vi "CT_DischargeEntryCleanup.vi"(2 "Load Number":i32, 3 "Cap Discharge Array In":T1=[{"cap number and switch SN array"=[{"Switch SN"="SN_U", "Cap Number"=109.0}], "Rog"=enum."F240", "Delay"=enum."PreForm", "Power Supply"=enum."PS1"}, {"cap number and switch SN array"=[{"Switch SN"="SN_U", "Cap Number"=110.0}], "Rog"=enum."F180", "Delay"=enum."DB16", "Power Supply"=enum."PS2"}, {"cap number and switch SN array"=[{"Switch SN"="SN_U", "Cap Number"=111.0}], "Rog"=enum."F300", "Delay"=enum."DB16", "Power Supply"=enum."PS2"}, {"cap number and switch SN array"=[{"Switch SN"="SN_U", "Cap Number"=112.0}], "Rog"=enum."F000", "Delay"=enum."DB16", "Power Supply"=enum."PS2"}, {"cap number and switch SN array"=[{"Switch SN"="SN_U", "Cap Number"=113.0}], "Rog"=enum."F060", "Delay"=enum."DB16", "Power Supply"=enum."PS2"}, {"cap number and switch SN array"=[{"Switch SN"="SN_U", "Cap Number"=114.0}], "Rog"=enum."F120", "Delay"=enum."DB16", "Power Supply"=enum."PS2"}, {"cap number and switch SN array"=[{"Switch SN"="SN_U", "Cap Number"=115.0}], "Rog"=enum."F120", "Delay"=enum."DB16", "Power Supply"=enum."PS2"}, {"cap number and switch SN array"=[{"Switch SN"="SN_U", "Cap Number"=116.0}], "Rog"=enum."F060", "Delay"=enum."DB16", "Power Supply"=enum."PS2"}, {"cap number and switch SN array"=[{"Switch SN"="SN_U", "Cap Number"=117.0}], "Rog"=enum."F000", "Delay"=enum."DB16", "Power Supply"=enum."PS2"}, {"cap number and switch SN array"=[{"Switch SN"="SN_U", "Cap Number"=118.0}], "Rog"=enum."F300", "Delay"=enum."DB16", "Power Supply"=enum."PS2"}, {"cap number and switch SN array"=[{"Switch SN"="SN_U", "Cap Number"=119.0}], "Rog"=enum."F180", "Delay"=enum."DB16", "Power Supply"=enum."PS2"}, {"cap number and switch SN array"=[{"Switch SN"="SN_U", "Cap Number"=120.0}], "Rog"=enum."F240", "Delay"=enum."DB16", "Power Supply"=enum."PS2"}, {"cap number and switch SN array"=[{"Switch SN"="SN_U", "Cap Number"=121.0}], "Rog"=enum."F240", "Delay"=enum."DB16", "Power Supply"=enum."PS3"}, {"cap number and switch SN array"=[{"Switch SN"="SN_U", "Cap Number"=122.0}], "Rog"=enum."F300", "Delay"=enum."DB16", "Power Supply"=enum."PS3"}, {"cap number and switch SN array"=[{"Switch SN"="SN_U", "Cap Number"=123.0}], "Rog"=enum."F180", "Delay"=enum."DB16", "Power Supply"=enum."PS3"}, {"cap number and switch SN array"=[{"Switch SN"="SN_U", "Cap Number"=124.0}], "Rog"=enum."F240", "Delay"=enum."DB16", "Power Supply"=enum."PS3"}, {"cap number and switch SN array"=[{"Switch SN"="SN_U", "Cap Number"=125.0}], "Rog"=enum."DISC", "Delay"=enum."DB16", "Power Supply"=enum."PS3"}, {"cap number and switch SN array"=[{"Switch SN"="SN_U", "Cap Number"=126.0}], "Rog"=enum."F000", "Delay"=enum."DB16", "Power Supply"=enum."PS3"}, {"cap number and switch SN array"=[{"Switch SN"="SN_U", "Cap Number"=127.0}], "Rog"=enum."F060", "Delay"=enum."DB16", "Power Supply"=enum."PS3"}, {"cap number and switch SN array"=[{"Switch SN"="SN_U", "Cap Number"=128.0}], "Rog"=enum."DISC", "Delay"=enum."DB16", "Power Supply"=enum."PS3"}]) -> (0 "Index of Module":u32, 1 "Cap Discharge Array Out":T1=[{"cap number and switch SN array"=[{"Switch SN"="SN_U", "Cap Number"=109.0}], "Rog"=enum."F240", "Delay"=enum."PreForm", "Power Supply"=enum."PS1"}, {"cap number and switch SN array"=[{"Switch SN"="SN_U", "Cap Number"=110.0}], "Rog"=enum."F180", "Delay"=enum."DB16", "Power Supply"=enum."PS2"}, {"cap number and switch SN array"=[{"Switch SN"="SN_U", "Cap Number"=111.0}], "Rog"=enum."F300", "Delay"=enum."DB16", "Power Supply"=enum."PS2"}, {"cap number and switch SN array"=[{"Switch SN"="SN_U", "Cap Number"=112.0}], "Rog"=enum."F000", "Delay"=enum."DB16", "Power Supply"=enum."PS2"}, {"cap number and switch SN array"=[{"Switch SN"="SN_U", "Cap Number"=113.0}], "Rog"=enum."F060", "Delay"=enum."DB16", "Power Supply"=enum."PS2"}, {"cap number and switch SN array"=[{"Switch SN"="SN_U", "Cap Number"=114.0}], "Rog"=enum."F120", "Delay"=enum."DB16", "Power Supply"=enum."PS2"}, {"cap number and switch SN array"=[{"Switch SN"="SN_U", "Cap Number"=115.0}], "Rog"=enum."F120", "Delay"=enum."DB16", "Power Supply"=enum."PS2"}, {"cap number and switch SN array"=[{"Switch SN"="SN_U", "Cap Number"=116.0}], "Rog"=enum."F060", "Delay"=enum."DB16", "Power Supply"=enum."PS2"}, {"cap number and switch SN array"=[{"Switch SN"="SN_U", "Cap Number"=117.0}], "Rog"=enum."F000", "Delay"=enum."DB16", "Power Supply"=enum."PS2"}, {"cap number and switch SN array"=[{"Switch SN"="SN_U", "Cap Number"=118.0}], "Rog"=enum."F300", "Delay"=enum."DB16", "Power Supply"=enum."PS2"}, {"cap number and switch SN array"=[{"Switch SN"="SN_U", "Cap Number"=119.0}], "Rog"=enum."F180", "Delay"=enum."DB16", "Power Supply"=enum."PS2"}, {"cap number and switch SN array"=[{"Switch SN"="SN_U", "Cap Number"=120.0}], "Rog"=enum."F240", "Delay"=enum."DB16", "Power Supply"=enum."PS2"}, {"cap number and switch SN array"=[{"Switch SN"="SN_U", "Cap Number"=121.0}], "Rog"=enum."F240", "Delay"=enum."DB16", "Power Supply"=enum."PS3"}, {"cap number and switch SN array"=[{"Switch SN"="SN_U", "Cap Number"=122.0}], "Rog"=enum."F300", "Delay"=enum."DB16", "Power Supply"=enum."PS3"}, {"cap number and switch SN array"=[{"Switch SN"="SN_U", "Cap Number"=123.0}], "Rog"=enum."F180", "Delay"=enum."DB16", "Power Supply"=enum."PS3"}, {"cap number and switch SN array"=[{"Switch SN"="SN_U", "Cap Number"=124.0}], "Rog"=enum."F240", "Delay"=enum."DB16", "Power Supply"=enum."PS3"}, {"cap number and switch SN array"=[{"Switch SN"="SN_U", "Cap Number"=125.0}], "Rog"=enum."DISC", "Delay"=enum."DB16", "Power Supply"=enum."PS3"}, {"cap number and switch SN array"=[{"Switch SN"="SN_U", "Cap Number"=126.0}], "Rog"=enum."F000", "Delay"=enum."DB16", "Power Supply"=enum."PS3"}, {"cap number and switch SN array"=[{"Switch SN"="SN_U", "Cap Number"=127.0}], "Rog"=enum."F060", "Delay"=enum."DB16", "Power Supply"=enum."PS3"}, {"cap number and switch SN array"=[{"Switch SN"="SN_U", "Cap Number"=128.0}], "Rog"=enum."DISC", "Delay"=enum."DB16", "Power Supply"=enum."PS3"}])   [LabVIEW 2016]
uses:
  CapDischargeCluster.ctl
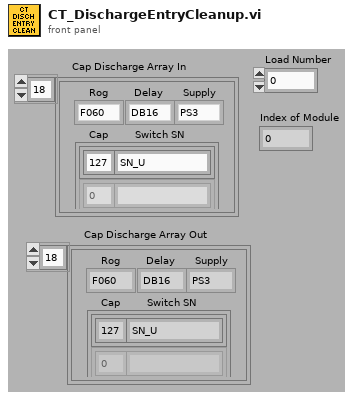
[diagram p1: front panel]
types:
  T1 = typedef "CapDischargeCluster.ctl" = cluster{"cap number and switch SN array":cluster{"Switch SN":string, "Cap Number":dbl}[], "Rog":enum16{"F000", "F060", "F120", "F180", "F240", "F300", "A015", "A045", "A075", "A105", "A135", "A165", "A195", "A225", "A255", "A285", "A315", "A345", "Snip", "DISC"}, "Delay":enum16{"DB00", "DB01", "DB02", "DB03", "DB04", "DB05", "DB06", "DB07", "DB08", "DB09", "DB10", "DB11", "DB12", "DB13", "DB14", "DB15", "DB16", "DB17", "DB18", "DB19", "DB20", "DB21", "DB22", "DB23", "DB24", "DB25", "DB26", "DB27", "DB28", "DB29", "DB30", "PreForm", "Form"}, "Power Supply":enum16{"PS1", "PS2", "PS3", "PS5", "PS6", "PS4"}}[]
  T2 = cluster{"cap number and switch SN array":cluster{"Switch SN":string, "Cap Number":dbl}[], "Rog":enum16{"F000", "F060", "F120", "F180", "F240", "F300", "A015", "A045", "A075", "A105", "A135", "A165", "A195", "A225", "A255", "A285", "A315", "A345", "Snip", "DISC"}, "Delay":enum16{"DB00", "DB01", "DB02", "DB03", "DB04", "DB05", "DB06", "DB07", "DB08", "DB09", "DB10", "DB11", "DB12", "DB13", "DB14", "DB15", "DB16", "DB17", "DB18", "DB19", "DB20", "DB21", "DB22", "DB23", "DB24", "DB25", "DB26", "DB27", "DB28", "DB29", "DB30", "PreForm", "Form"}, "Power Supply":enum16{"PS1", "PS2", "PS3", "PS5", "PS6", "PS4"}}
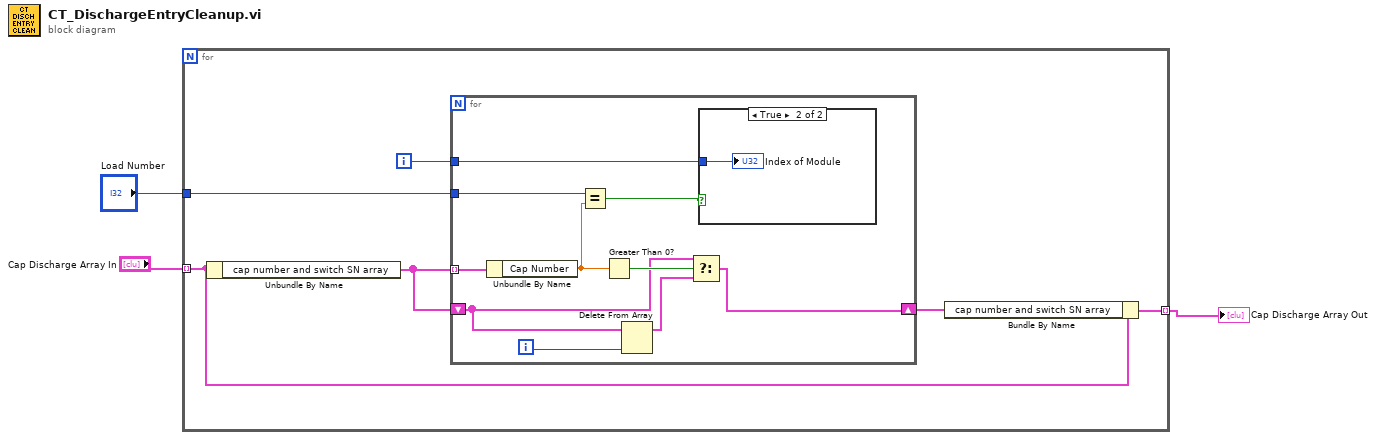
[diagram p0: block diagram]
diagram:
  n1 = for {
    tunnel: "Cap Discharge Array In" -> [w8] mode=indexing
    tunnel: [w6] -> w1 mode=indexing
    tunnel: "Load Number" -> [w5]
    i -> [w4]
    n2 = Unbundle By Name(w8) -> ("cap number and switch SN array"=w9:cluster{"Switch SN":string, "Cap Number":dbl}[])
    n3 = for {
      tunnel: w9 -> [w19] mode=indexing
      shift-right: [w17] -> w7
      shift-left: w9 -> [w16]
      tunnel: w5 -> [w12]
      tunnel: w4 -> [w10]
      i -> [w15]
      n4 = Unbundle By Name(w19) -> ("Cap Number"=w13:dbl)
      n5 = Equal?(x=w12, y=w13) -> (x = y?=w11:bool)
      n6 = Greater Than 0?(x=w13) -> (x > 0?=w18:bool)
      n7 = Delete From Array(array=w16, index=w15) -> (array with subset deleted=w14:cluster{"Switch SN":string, "Cap Number":dbl}[])  [unwired: 1 in, 1 out]
      n8 = Select(t=w16, s=w18, f=w14) -> (s? t:f=w17:cluster{"Switch SN":string, "Cap Number":dbl}[])
      n9 = case shown="True" w11 {
        tunnel: w10 -> [_ w20]
        frame False {
        }
        frame True {
          "Index of Module" <- w20
        }
      }
    }
    n10 = Bundle By Name(cluster=w8, "cap number and switch SN array"=w7) -> (w6:T2)
  }
  "Cap Discharge Array Out" <- w1
